vi "Temp Control Final Product.vi"() -> ()   [LabVIEW 2021]
doc: "This example demonstrates temperature control and monitoring.\n\nNote:\nBefore start this VI is it necessary:\n- allowed used blocks in Instrument Options (by Eurotherm iTools or by instrument front panel controls)\n- preconfigured some specific parameters this are not supported by this driver (e.g. PV-I/O Type, Linearization type, Alarm Input Values... ) by Eurotherm iTools or by instrument front panel controls\n- enter correct VISA Resource Descriptor and Device Address into front-panel controls"
uses:
  Eurotherm 35xx Series.lvlib
panel:
  in  "Dwell time (mins)":u32
  in  "Initial temp":i32
  in  "End Temp":i32
  in  "Goal Temp":i32
  in  "stop":bool
  in  "Unit Address (1)":u8=1
  in  "VISA resource name":refnum<visa-resource-name>
  # "There are two goal temps because of the case \nstructure- one goal temp for ramp up (ex:500)\none end temp for ramp down (ex: 0)"
  # "(c) 2005-2010 NATIONAL INSTRUMENTS.  ALL RIGHTS RESERVED."
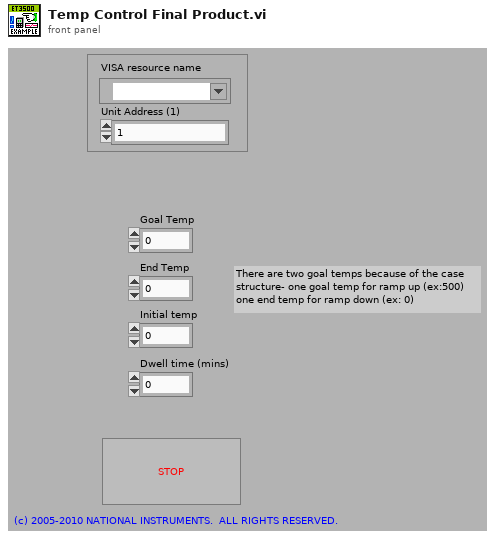
[diagram p1: front panel]
types:
  T1 = cluster{"Baud Rate (19200)":u32, "Parity (0: None)":u16, "Break Length (0)":u16}
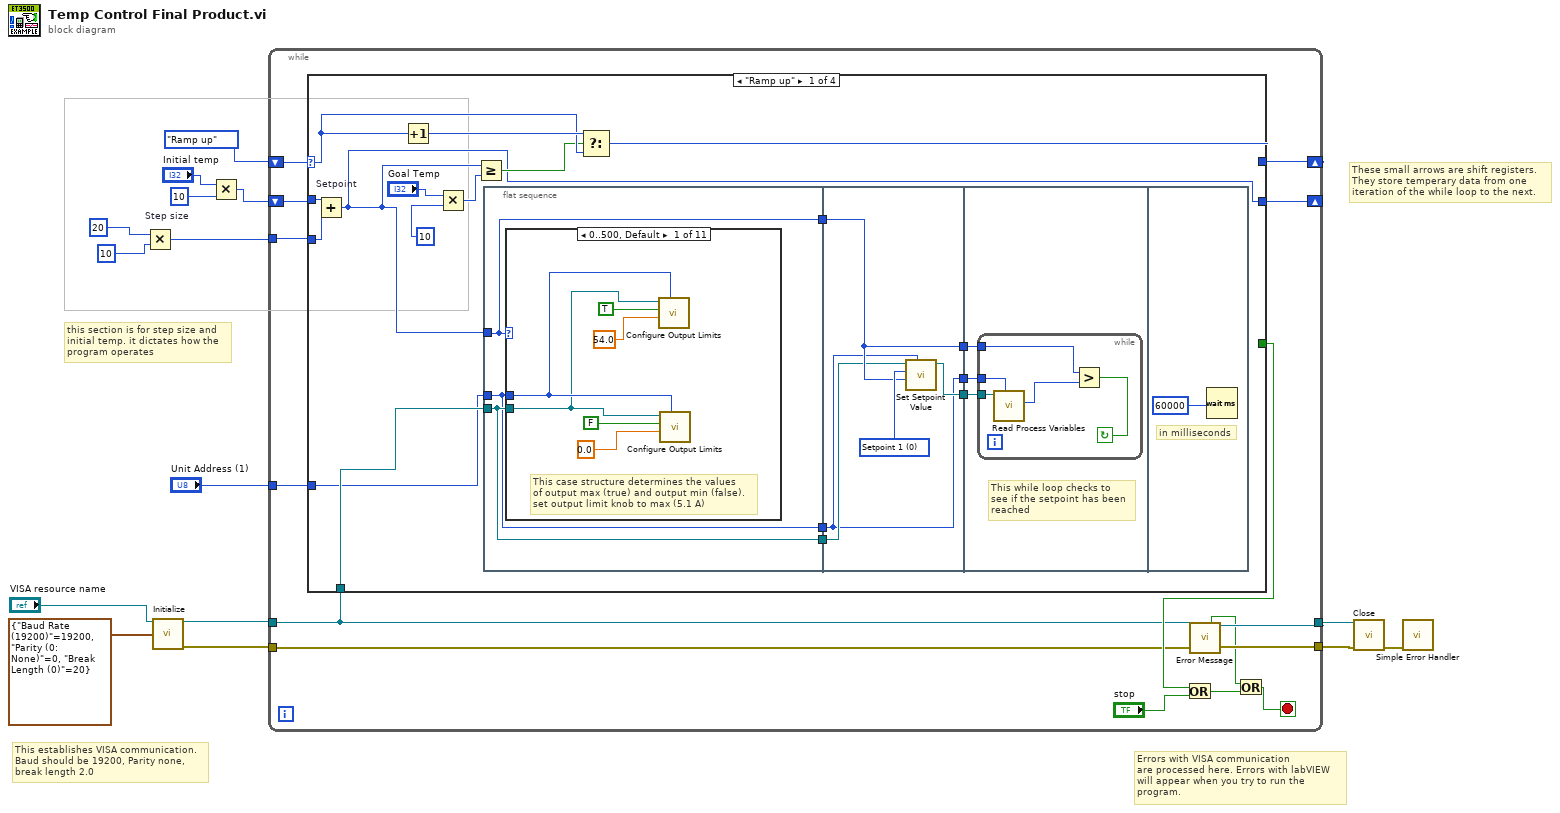
[diagram p0: block diagram]
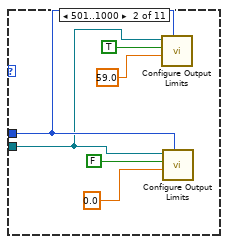
[diagram p2: hidden frame]
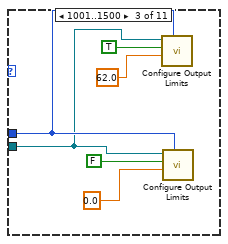
[diagram p3: hidden frame]
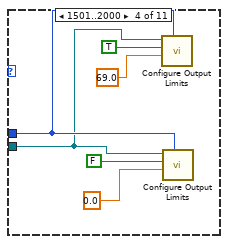
[diagram p4: hidden frame]
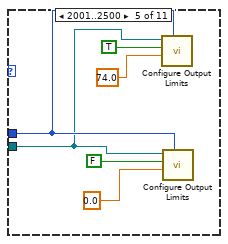
[diagram p5: hidden frame]
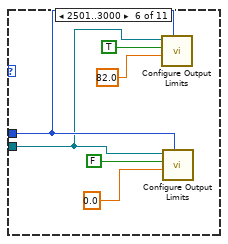
[diagram p6: hidden frame]
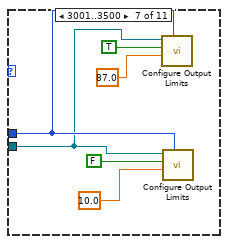
[diagram p7: hidden frame]
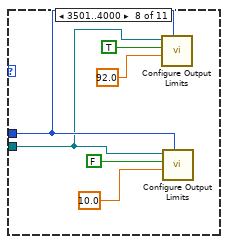
[diagram p8: hidden frame]
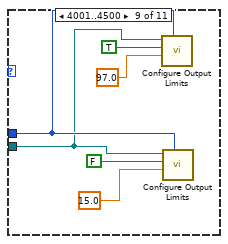
[diagram p9: hidden frame]
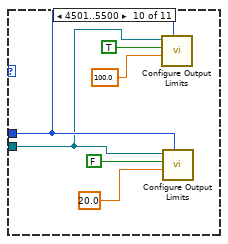
[diagram p10: hidden frame]
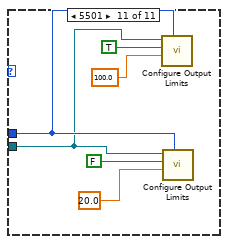
[diagram p11: hidden frame]
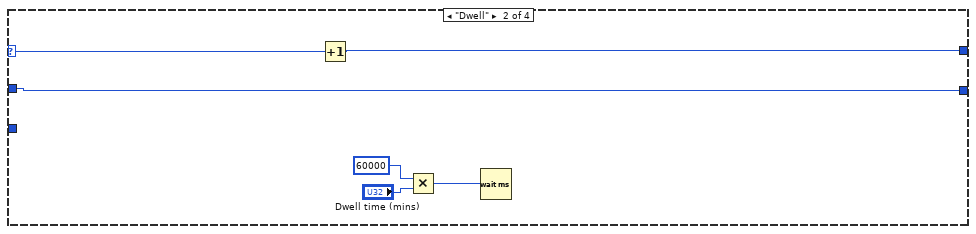
[diagram p12: hidden frame]
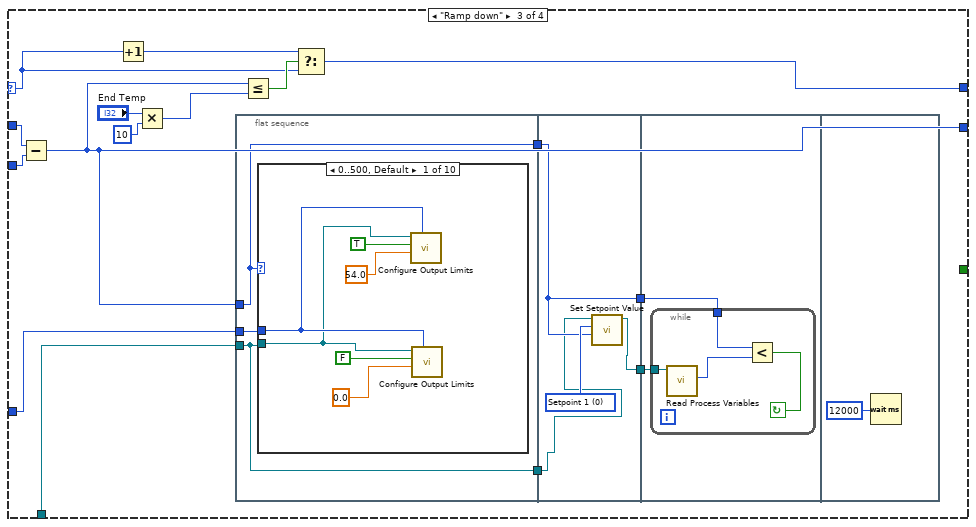
[diagram p13: hidden frame]
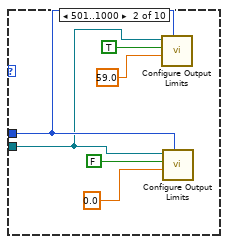
[diagram p14: hidden frame]
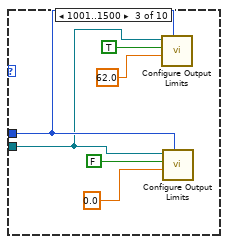
[diagram p15: hidden frame]
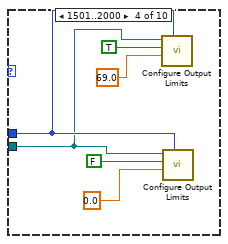
[diagram p16: hidden frame]
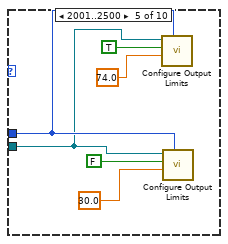
[diagram p17: hidden frame]
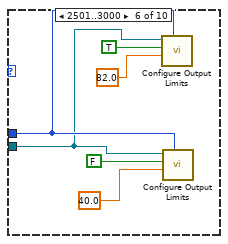
[diagram p18: hidden frame]
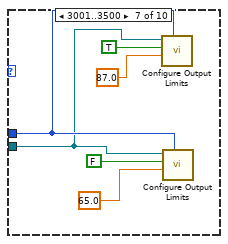
[diagram p19: hidden frame]
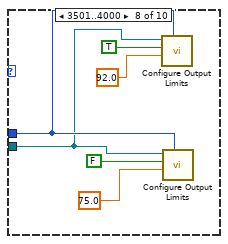
[diagram p20: hidden frame]
diagram:
  # "These small arrows are shift registers.\nThey store temperary data from one \niteration of the while loop to the next."
  # "Errors with VISA communication \nare processed here. Errors with labVIEW \nwill appear when you try to run the \nprogram."
  # "This establishes VISA communication.\nBaud should be 19200, Parity none, \nbreak length 2.0"
  # "this section is for step size and \ninitial temp. it dictates how the \nprogram operates"
  n1 = Multiply "Step size"(x=20, y=10) -> (x*y=w8:i32)
  n2 = call "Initialize.vi"("VISA resource name"="VISA resource name", "Serial Configuration"=T1 {"Baud Rate (19200)"=19200, "Parity (0: None)"=0, "Break Length (0)"=20}) -> ("VISA resource name out"=w6:refnum<visa-resource-name>, "error out"=w5:errorcluster)  [unwired: 12 in]
  n3 = Multiply(x="Initial temp", y=10) -> (x*y=w3:i32)
  n4 = while {
    tunnel: w6 -> [w17]
    tunnel: w5 -> [w16]
    tunnel: "Unit Address (1)" -> [w18]
    tunnel: [w30] -> w12
    tunnel: [w29] -> w13
    tunnel: w8 -> [w25]
    shift-right: [w24] -> _
    shift-left: enum16{"Ramp up", "Dwell", "Ramp down", "Stop"}."Ramp up" ("should be a typedef") -> [w26]
    shift-right: [w20] -> _
    shift-left: w3 -> [w19]
    stop <- w28 stop-if-true
    n5 = case shown="\"Ramp up\"" w26 {
      selector: w26 -> [w46 w137 w146 _]
      tunnel: [w45 w135 w147 _] -> w24
      tunnel: [_ _ _ TRUE] -> w23
      tunnel: [w39 w136 w143 w228] -> w20
      tunnel: w19 -> [w48 w136 w148 w228]
      tunnel: w25 -> [w43 _ w149 _]
      tunnel: w18 -> [w37 _ w144 _]
      tunnel: w17 -> [w38 _ w142 _]
      frame "Ramp up" {
        n6 = Add "Setpoint"(x=w48, y=w43) -> (x+y=w39:i32)
        n7 = Increment(x=w46) -> (x+1=w47:enum16{"Ramp up", "Dwell", "Ramp down", "Stop"})
        n8 = Multiply(x="Goal Temp", y=10) -> (x*y=w42:i32)
        n9 = Greater Or Equal?(x=w39, y=w42) -> (x >= y?=w44:bool)
        n10 = flat-sequence {
          tunnel: w39 -> [w51]
          tunnel: w38 -> [w50]
          tunnel: w37 -> [w49]
          tunnel: [w51] -> w35
          tunnel: [w50] -> w33
          tunnel: [w49] -> w32
          tunnel: [w121] -> w36
          tunnel: w35 -> [w120]
          tunnel: [w120] -> w34
          tunnel: w33 -> [w119]
          tunnel: w32 -> [w118]
          tunnel: [w118] -> w31
          tunnel: w36 -> [w125]
          tunnel: w34 -> [w124]
          tunnel: w31 -> [w123]
          frame #0 {
            n11 = case shown="0..500, Default" w51 {
              tunnel: w49 -> [w53 w59 w65 w71 w77 w83 w89 w95 w101 w107 w113]
              tunnel: w50 -> [w52 w58 w64 w70 w76 w82 w88 w94 w100 w106 w112]
              frame 0..500, Default {
                # "This case structure determines the values\nof output max (true) and output min (false).\nset output limit knob to max (5.1 A)"
                n12 = call "Configure Output Limits.vi"("Unit Address (1)"=w53, "Output Limit Value (0)"=sgl 54.0, "Enable Limit Type  (False: Low)"=TRUE, "VISA resource name"=w52) -> ()  [unwired: 6 in, 2 out]
                n13 = call "Configure Output Limits.vi"("Unit Address (1)"=w53, "Output Limit Value (0)"=sgl 0.0, "Enable Limit Type  (False: Low)"=FALSE, "VISA resource name"=w52) -> ()  [unwired: 6 in, 2 out]
              }
              frame 501..1000 {
                n14 = call "Configure Output Limits.vi"("Unit Address (1)"=w59, "Output Limit Value (0)"=sgl 59.0, "Enable Limit Type  (False: Low)"=TRUE, "VISA resource name"=w58) -> ()  [unwired: 6 in, 2 out]
                n15 = call "Configure Output Limits.vi"("Unit Address (1)"=w59, "Output Limit Value (0)"=sgl 0.0, "Enable Limit Type  (False: Low)"=FALSE, "VISA resource name"=w58) -> ()  [unwired: 6 in, 2 out]
              }
              frame 1001..1500 {
                n16 = call "Configure Output Limits.vi"("Unit Address (1)"=w65, "Output Limit Value (0)"=sgl 62.0, "Enable Limit Type  (False: Low)"=TRUE, "VISA resource name"=w64) -> ()  [unwired: 6 in, 2 out]
                n17 = call "Configure Output Limits.vi"("Unit Address (1)"=w65, "Output Limit Value (0)"=sgl 0.0, "Enable Limit Type  (False: Low)"=FALSE, "VISA resource name"=w64) -> ()  [unwired: 6 in, 2 out]
              }
              frame 1501..2000 {
                n18 = call "Configure Output Limits.vi"("Unit Address (1)"=w71, "Output Limit Value (0)"=sgl 69.0, "Enable Limit Type  (False: Low)"=TRUE, "VISA resource name"=w70) -> ()  [unwired: 6 in, 2 out]
                n19 = call "Configure Output Limits.vi"("Unit Address (1)"=w71, "Output Limit Value (0)"=sgl 0.0, "Enable Limit Type  (False: Low)"=FALSE, "VISA resource name"=w70) -> ()  [unwired: 6 in, 2 out]
              }
              frame 2001..2500 {
                n20 = call "Configure Output Limits.vi"("Unit Address (1)"=w77, "Output Limit Value (0)"=sgl 74.0, "Enable Limit Type  (False: Low)"=TRUE, "VISA resource name"=w76) -> ()  [unwired: 6 in, 2 out]
                n21 = call "Configure Output Limits.vi"("Unit Address (1)"=w77, "Output Limit Value (0)"=sgl 0.0, "Enable Limit Type  (False: Low)"=FALSE, "VISA resource name"=w76) -> ()  [unwired: 6 in, 2 out]
              }
              frame 2501..3000 {
                n22 = call "Configure Output Limits.vi"("Unit Address (1)"=w83, "Output Limit Value (0)"=sgl 82.0, "Enable Limit Type  (False: Low)"=TRUE, "VISA resource name"=w82) -> ()  [unwired: 6 in, 2 out]
                n23 = call "Configure Output Limits.vi"("Unit Address (1)"=w83, "Output Limit Value (0)"=sgl 0.0, "Enable Limit Type  (False: Low)"=FALSE, "VISA resource name"=w82) -> ()  [unwired: 6 in, 2 out]
              }
              frame 3001..3500 {
                n24 = call "Configure Output Limits.vi"("Unit Address (1)"=w89, "Output Limit Value (0)"=sgl 87.0, "Enable Limit Type  (False: Low)"=TRUE, "VISA resource name"=w88) -> ()  [unwired: 6 in, 2 out]
                n25 = call "Configure Output Limits.vi"("Unit Address (1)"=w89, "Output Limit Value (0)"=sgl 10.0, "Enable Limit Type  (False: Low)"=FALSE, "VISA resource name"=w88) -> ()  [unwired: 6 in, 2 out]
              }
              frame 3501..4000 {
                n26 = call "Configure Output Limits.vi"("Unit Address (1)"=w95, "Output Limit Value (0)"=sgl 92.0, "Enable Limit Type  (False: Low)"=TRUE, "VISA resource name"=w94) -> ()  [unwired: 6 in, 2 out]
                n27 = call "Configure Output Limits.vi"("Unit Address (1)"=w95, "Output Limit Value (0)"=sgl 10.0, "Enable Limit Type  (False: Low)"=FALSE, "VISA resource name"=w94) -> ()  [unwired: 6 in, 2 out]
              }
              frame 4001..4500 {
                n28 = call "Configure Output Limits.vi"("Unit Address (1)"=w101, "Output Limit Value (0)"=sgl 97.0, "Enable Limit Type  (False: Low)"=TRUE, "VISA resource name"=w100) -> ()  [unwired: 6 in, 2 out]
                n29 = call "Configure Output Limits.vi"("Unit Address (1)"=w101, "Output Limit Value (0)"=sgl 15.0, "Enable Limit Type  (False: Low)"=FALSE, "VISA resource name"=w100) -> ()  [unwired: 6 in, 2 out]
              }
              frame 4501..5500 {
                n30 = call "Configure Output Limits.vi"("Unit Address (1)"=w107, "Output Limit Value (0)"=sgl 100.0, "Enable Limit Type  (False: Low)"=TRUE, "VISA resource name"=w106) -> ()  [unwired: 6 in, 2 out]
                n31 = call "Configure Output Limits.vi"("Unit Address (1)"=w107, "Output Limit Value (0)"=sgl 20.0, "Enable Limit Type  (False: Low)"=FALSE, "VISA resource name"=w106) -> ()  [unwired: 6 in, 2 out]
              }
              frame 5501 {
                n32 = call "Configure Output Limits.vi"("Unit Address (1)"=w113, "Output Limit Value (0)"=sgl 100.0, "Enable Limit Type  (False: Low)"=TRUE, "VISA resource name"=w112) -> ()  [unwired: 6 in, 2 out]
                n33 = call "Configure Output Limits.vi"("Unit Address (1)"=w113, "Output Limit Value (0)"=sgl 20.0, "Enable Limit Type  (False: Low)"=FALSE, "VISA resource name"=w112) -> ()  [unwired: 6 in, 2 out]
              }
            }
          }
          frame #1 {
            w122 = u8 0 items=["Setpoint 1", "Setpoint 2", "Alternate Setpoint", "Target Setpoint"] ("Selected Setpoint (0: Setpoint 1)")
            n34 = call "Set Setpoint Value.vi"("Unit Address (1)"=w118, "Setpoint Value (0)"=w120, "Selected Setpoint (0: Setpoint 1)"=w122, "VISA resource name"=w119) -> ("VISA resource name out"=w121:refnum<visa-resource-name>)  [unwired: 6 in, 1 out]
          }
          frame #2 {
            # "This while loop checks to \nsee if the setpoint has been\nreached"
            n35 = while {
              tunnel: w125 -> [w128]
              tunnel: w124 -> [w127]
              tunnel: w123 -> [w126]
              stop <- w129 continue-if-true
              n36 = call "Read Process Variables.vi"("Unit Address (1)"=w126, "VISA resource name"=w128) -> ("Process Value"=w130:i16)  [unwired: 6 in, 3 out]
              n37 = Greater?(x=w127, y=w130) -> (0:w129:bool)
            }
          }
          frame #3 {
            # "in milliseconds"
            n38 = Wait (ms)(milliseconds to wait=u32 60000 ("millisecond timer value")) -> ()  [unwired: 1 out]
          }
        }
        n39 = Select(t=w47, s=w44, f=w46) -> (s? t:f=w45:enum16{"Ramp up", "Dwell", "Ramp down", "Stop"})
      }
      frame "Dwell" {
        n40 = Increment(x=w137) -> (x+1=w135:enum16{"Ramp up", "Dwell", "Ramp down", "Stop"})
        n41 = Multiply(x=u32 60000, y="Dwell time (mins)") -> (x*y=w133:u32)
        n42 = Wait (ms)(milliseconds to wait=w133) -> ()  [unwired: 1 out]
      }
      frame "Ramp down" {
        n43 = Subtract(x=w148, y=w149) -> (x-y=w143:i32)
        n44 = Increment(x=w146) -> (x+1=w153:enum16{"Ramp up", "Dwell", "Ramp down", "Stop"})
        n45 = Multiply(x="End Temp", y=10) -> (x*y=w151:i32)
        n46 = flat-sequence {
          tunnel: w144 -> [w156]
          tunnel: w143 -> [w155]
          tunnel: w142 -> [w154]
          tunnel: [w155] -> w140
          tunnel: [w154] -> w138
          tunnel: [w219] -> w141
          tunnel: w140 -> [w218]
          tunnel: [w218] -> w139
          tunnel: w138 -> [w217]
          tunnel: w141 -> [w222]
          tunnel: w139 -> [w221]
          frame #0 {
            n47 = case shown="0..500, Default" w155 {
              tunnel: w156 -> [w158 w164 w170 w176 w182 w188 w194 w200 w206 w212]
              tunnel: w154 -> [w157 w163 w169 w175 w181 w187 w193 w199 w205 w211]
              frame 0..500, Default {
                n48 = call "Configure Output Limits.vi"("Unit Address (1)"=w158, "Output Limit Value (0)"=sgl 54.0, "Enable Limit Type  (False: Low)"=TRUE, "VISA resource name"=w157) -> ()  [unwired: 6 in, 2 out]
                n49 = call "Configure Output Limits.vi"("Unit Address (1)"=w158, "Output Limit Value (0)"=sgl 0.0, "Enable Limit Type  (False: Low)"=FALSE, "VISA resource name"=w157) -> ()  [unwired: 6 in, 2 out]
              }
              frame 501..1000 {
                n50 = call "Configure Output Limits.vi"("Unit Address (1)"=w164, "Output Limit Value (0)"=sgl 59.0, "Enable Limit Type  (False: Low)"=TRUE, "VISA resource name"=w163) -> ()  [unwired: 6 in, 2 out]
                n51 = call "Configure Output Limits.vi"("Unit Address (1)"=w164, "Output Limit Value (0)"=sgl 0.0, "Enable Limit Type  (False: Low)"=FALSE, "VISA resource name"=w163) -> ()  [unwired: 6 in, 2 out]
              }
              frame 1001..1500 {
                n52 = call "Configure Output Limits.vi"("Unit Address (1)"=w170, "Output Limit Value (0)"=sgl 62.0, "Enable Limit Type  (False: Low)"=TRUE, "VISA resource name"=w169) -> ()  [unwired: 6 in, 2 out]
                n53 = call "Configure Output Limits.vi"("Unit Address (1)"=w170, "Output Limit Value (0)"=sgl 0.0, "Enable Limit Type  (False: Low)"=FALSE, "VISA resource name"=w169) -> ()  [unwired: 6 in, 2 out]
              }
              frame 1501..2000 {
                n54 = call "Configure Output Limits.vi"("Unit Address (1)"=w176, "Output Limit Value (0)"=sgl 69.0, "Enable Limit Type  (False: Low)"=TRUE, "VISA resource name"=w175) -> ()  [unwired: 6 in, 2 out]
                n55 = call "Configure Output Limits.vi"("Unit Address (1)"=w176, "Output Limit Value (0)"=sgl 0.0, "Enable Limit Type  (False: Low)"=FALSE, "VISA resource name"=w175) -> ()  [unwired: 6 in, 2 out]
              }
              frame 2001..2500 {
                n56 = call "Configure Output Limits.vi"("Unit Address (1)"=w182, "Output Limit Value (0)"=sgl 74.0, "Enable Limit Type  (False: Low)"=TRUE, "VISA resource name"=w181) -> ()  [unwired: 6 in, 2 out]
                n57 = call "Configure Output Limits.vi"("Unit Address (1)"=w182, "Output Limit Value (0)"=sgl 30.0, "Enable Limit Type  (False: Low)"=FALSE, "VISA resource name"=w181) -> ()  [unwired: 6 in, 2 out]
              }
              frame 2501..3000 {
                n58 = call "Configure Output Limits.vi"("Unit Address (1)"=w188, "Output Limit Value (0)"=sgl 82.0, "Enable Limit Type  (False: Low)"=TRUE, "VISA resource name"=w187) -> ()  [unwired: 6 in, 2 out]
                n59 = call "Configure Output Limits.vi"("Unit Address (1)"=w188, "Output Limit Value (0)"=sgl 40.0, "Enable Limit Type  (False: Low)"=FALSE, "VISA resource name"=w187) -> ()  [unwired: 6 in, 2 out]
              }
              frame 3001..3500 {
                n60 = call "Configure Output Limits.vi"("Unit Address (1)"=w194, "Output Limit Value (0)"=sgl 87.0, "Enable Limit Type  (False: Low)"=TRUE, "VISA resource name"=w193) -> ()  [unwired: 6 in, 2 out]
                n61 = call "Configure Output Limits.vi"("Unit Address (1)"=w194, "Output Limit Value (0)"=sgl 65.0, "Enable Limit Type  (False: Low)"=FALSE, "VISA resource name"=w193) -> ()  [unwired: 6 in, 2 out]
              }
              frame 3501..4000 {
                n62 = call "Configure Output Limits.vi"("Unit Address (1)"=w200, "Output Limit Value (0)"=sgl 92.0, "Enable Limit Type  (False: Low)"=TRUE, "VISA resource name"=w199) -> ()  [unwired: 6 in, 2 out]
                n63 = call "Configure Output Limits.vi"("Unit Address (1)"=w200, "Output Limit Value (0)"=sgl 75.0, "Enable Limit Type  (False: Low)"=FALSE, "VISA resource name"=w199) -> ()  [unwired: 6 in, 2 out]
              }
              frame 4001..4500 {
                n64 = call "Configure Output Limits.vi"("Unit Address (1)"=w206, "Output Limit Value (0)"=sgl 97.0, "Enable Limit Type  (False: Low)"=TRUE, "VISA resource name"=w205) -> ()  [unwired: 6 in, 2 out]
                n65 = call "Configure Output Limits.vi"("Unit Address (1)"=w206, "Output Limit Value (0)"=sgl 80.0, "Enable Limit Type  (False: Low)"=FALSE, "VISA resource name"=w205) -> ()  [unwired: 6 in, 2 out]
              }
              frame 4501..5500 {
                n66 = call "Configure Output Limits.vi"("Unit Address (1)"=w212, "Output Limit Value (0)"=sgl 100.0, "Enable Limit Type  (False: Low)"=TRUE, "VISA resource name"=w211) -> ()  [unwired: 6 in, 2 out]
                n67 = call "Configure Output Limits.vi"("Unit Address (1)"=w212, "Output Limit Value (0)"=sgl 90.0, "Enable Limit Type  (False: Low)"=FALSE, "VISA resource name"=w211) -> ()  [unwired: 6 in, 2 out]
              }
            }
          }
          frame #1 {
            w220 = u8 0 items=["Setpoint 1", "Setpoint 2", "Alternate Setpoint", "Target Setpoint"] ("Selected Setpoint (0: Setpoint 1)")
            n68 = call "Set Setpoint Value.vi"("Setpoint Value (0)"=w218, "Selected Setpoint (0: Setpoint 1)"=w220, "VISA resource name"=w217) -> ("VISA resource name out"=w219:refnum<visa-resource-name>)  [unwired: 7 in, 1 out]
          }
          frame #2 {
            n69 = while {
              tunnel: w222 -> [w224]
              tunnel: w221 -> [w223]
              stop <- w225 continue-if-true
              n70 = call "Read Process Variables.vi"("VISA resource name"=w224) -> ("Process Value"=w226:i16)  [unwired: 7 in, 3 out]
              n71 = Less?(x=w223, y=w226) -> (x < y?=w225:bool)
            }
          }
          frame #3 {
            n72 = Wait (ms)(milliseconds to wait=u32 12000 ("millisecond timer value")) -> ()  [unwired: 1 out]
          }
        }
        n73 = Less Or Equal?(x=w143, y=w151) -> (x <= y?=w152:bool)
        n74 = Select(t=w153, s=w152, f=w146) -> (s? t:f=w147:enum16{"Ramp up", "Dwell", "Ramp down", "Stop"})
      }
      frame "Stop" {
      }
    }
    n75 = Or(x=w23, y="stop") -> (x .or. y?=w21:bool)
    n76 = call "Error Message.vi"("VISA resource name"=w17, "error in (no error)"=w16) -> ("Status"=w27:bool, "VISA resource name out"=w30:refnum<visa-resource-name>, "error out"=w29:errorcluster)  [unwired: 9 in, 2 out]
    n77 = Or(x=w27, y=w21) -> (x .or. y?=w28:bool)
  }
  n78 = call "Close.vi"("VISA resource name"=w12, "error in (no error)"=w13) -> ("error out"=w11:errorcluster)  [unwired: 13 in]
  n79 = call <vilib>:"Simple Error Handler.vi"("error in (no error)"=w11) -> ()  [unwired: 4 in, 5 out]
